vi "Main.vi"() -> ()   [LabVIEW 2013] (continued)
                    n2203 = call "Msgbox - Message Handler.vi"("Short Description (When DB Not Available)"="WPS Details Incomplete" ("string"), "Description (When DB Not Available)"=" must be entered" ("string"), "Pre-Description"=w3600, "<.?....> Message Code"="<E 524>") -> ("MHandler Error"=w3599:errorcluster)  [unwired: 5 in, 2 out]
                    n2204 = local write "MHandler"(w3599) -> ()
                  }
                }
              }
            }
          }
          frame True {
            # "Incomplete Fields In Header"
            n2205 = control-ref of="WPS Details Master Data"() -> (w3634:refnum<vi>)
            n2206 = property class="Clust (strict)"(reference=w3634) -> ("Caption.Text"=w3630:string)  [unwired: 1 in, 2 out]
            n2207 = case shown="\"Master Data Delete\", Default" w3633 {
              tunnel: ["{Delete WPS}" ("string") "{Save WPS}" ("string")] -> _
              frame "Master Data Delete", Default {
                # "No longer available"
              }
              frame "Master Data Save" {
              }
            }
            n2208 = local read "Logon Extra"() -> (w3628:T25)
            n2209 = Unbundle By Name(w3628) -> ("IsUnicode"=w3627:bool)
            n2210 = call "String - Add BOM if IsUnicode.vi"("Input is Unicode (varbinary)?"=w3627, "String IN"=w3630) -> ("BOM Added"=w3629:string)  [unwired: 9 in]
            n2211 = call "Msgbox - Message Handler.vi"("Short Description (When DB Not Available)"=" WPS Details Incomplete", "Description (When DB Not Available)"=" must be entered." ("message"), "Pre-Description"=w3629, "<.?....> Message Code"="<E 524>") -> ("MHandler Error"=w3632:errorcluster)  [unwired: 5 in, 2 out]
            n2212 = local write "MHandler"(w3632) -> ()
          }
        }
      }
      event Mouse Down? {
        # "User Clicks on MasterData\\WPS ComboBox"
        n2213 = event-data() -> ("Time"=→"WPS Details Master Data: Mouse Down":u32, "CtlRef"=w3639:refnum<vi>)  [unwired: 1 in, 6 out]
        n2214 = case shown="True" "DB - Master Data Load" {
          tunnel: w3639 -> [w3642 w3646]
          frame False {
            # "List of wps found"
            # "<wps/ref>_<rev>.wps"
            # "<wps/ref>_<rev>.wps"
            # "Use .wps"
            n2215 = local read "MasterData\\WPS"() -> (w3645:path)
            n2216 = List Folder(path=w3645, pattern="*.wps") -> (filenames=w3641:string[])  [unwired: 2 in, 3 out]
            "Temp Array" <- w3641
            n2217 = call "String - Extract Unique Headers_.vi"("Array In"=w3641) -> ("Array Out"=w3643:string[])  [unwired: 10 in]
            n2218 = property class="CmbBox (strict)"(reference=w3642, "Strings[]"=w3643) -> ()  [unwired: 1 in, 2 out]
          }
          frame True {
            # "Use DB"
            n2219 = call "DB - [MasterData].[Procedure].vi"("DB - Master Data Enum"=DB_-_Master_Data_Procedure_Enum."SELECT [ProcedureNo]", "CmbBox Refnum"=w3646) -> ("SUMMARY"=w3647:errorcluster)  [unwired: 10 in, 3 out]
            n2220 = local write "DB"(w3647) -> ()
          }
        }
        n2221 = event-data() -> ()  [unwired: 2 in, 1 out]
      }
      event Value Change {
        # "<wps/ref>_<rev>.wps"
        n2222 = event-data() -> ("Time"=→"WPS Details Master Data: Value Change":u32, "CtlRef"=w3651:refnum<vi>)  [unwired: 1 in, 4 out]
        n2223 = local read "DB - Master Data Load"() -> (w3653:bool)
        n2224 = property class="CmbBox (strict)"(reference=w3651) -> ("Label.Text"=w3656:string, "Value"=w3654:T5)  [unwired: 1 in, 2 out]
        n2225 = case shown="\"WPS/Ref\", Default" w3656 {
          tunnel: [w3678 w3686 _] -> _
          tunnel: [w3677 w3685 _] -> _
          tunnel: [w3676 w3684 w3697] -> w3655
          tunnel: [w3675 w3683 _] -> _
          tunnel: w3654 -> [w3673 _ w3695]
          tunnel: [w3671 w3682 w3688] -> w3650
          tunnel: [w3670 w3681 w3687] -> w3649
          frame "WPS/Ref", Default {
            w3670 = FALSE  # Include Inactive
            # "Copies Value to Extra WPS\nHighlight Entire Text"
            n2226 = control-ref of="WPS Details Setup"() -> (w3671:refnum<vi>)
            n2227 = control-ref of="WPS/Ref"() -> ()  [unwired: 1 out]
            n2228 = control-ref of="Rev"() -> (w3676:refnum<vi>)
            n2229 = control-ref of="Hold Temperature"() -> (w3677:refnum<vi>)
            n2230 = control-ref of="Hold Time (HH:MM)"() -> (w3675:refnum<vi>)
            n2231 = control-ref of="MCListBox FHS Setup"() -> (w3678:refnum<vi>)
            n2232 = control-ref of="Extra WPS"() -> (w3674:refnum<vi>)
            n2233 = property on="Property Node" class="Str"(reference=w3674, "Value"=w3673) -> (error out=w3672:errorcluster)  [unwired: 1 in, 1 out]
            n2234 = flat-sequence {
              tunnel: w3672 -> [_]
              frame #0 {
                n2235 = property on="Extra WPS" class="Str"("Key Focus"=TRUE, "Text.Selection"=T58 {"Selection Start"=0, "Selection End"=100}) -> ()  [unwired: 2 in, 2 out]
              }
            }
          }
          frame "Master Data WPS/Ref" {
            w3681 = TRUE  # Include Inactive
            n2236 = control-ref of="WPS Details Master Data"() -> (w3682:refnum<vi>)
            n2237 = control-ref of="Master Data WPS/Ref"() -> ()  [unwired: 1 out]
            n2238 = control-ref of="Master Data Rev"() -> (w3684:refnum<vi>)
            n2239 = control-ref of="Master Data Hold Temperature"() -> (w3685:refnum<vi>)
            n2240 = control-ref of="Master Data Hold Time (HH:MM)"() -> (w3683:refnum<vi>)
            n2241 = control-ref of="MCListBox FHS Master Data"() -> (w3686:refnum<vi>)
          }
          frame "Additional WPS/Ref" {
            w3687 = FALSE  # Include Inactive
            w3696 = T13 {"Master Data WPS/Ref"="", "Master Data Rev"="", "Master Data Hold Temperature"="", "Master Data Temperature Units"="", "Master Data Hold Time (HH:MM)"="", "Inactive"=FALSE}  # Cluster
            # "to be implemented"
            n2242 = control-ref of="Additional Rev"() -> (w3697:refnum<vi>)
            n2243 = Bundle(cluster=w3696, "Master Data WPS/Ref"=w3695, "Master Data Rev"=T5 "", "Master Data Hold Temperature"="", "Master Data Temperature Units"="", "Master Data Hold Time (HH:MM)"="", "Inactive"=FALSE) -> (→"WPS Details Buffer (DB)":T13)
            n2244 = control-ref of="WPS Details Buffer (DB)"() -> (w3688:refnum<vi>)
          }
        }
        n2245 = case shown="True" w3653 {
          tunnel: w3655 -> [w3659 w3667]
          tunnel: w3654 -> [w3657 _]
          tunnel: w3650 -> [_ w3664]
          tunnel: w3649 -> [_ w3665]
          frame False {
            # "Show BLANK as Rev and update Details according to BLANK"
            n2246 = local read "Temp Array"() -> (w3661:string[])
            n2247 = call "String - Extract _Body_.vi"("Temp Array"=w3661, "<wps>"=w3657) -> ("<rev>"=w3660:string[])  [unwired: 9 in]
            n2248 = property on="Property Node" class="CmbBox (strict)"(reference=w3659, "Strings[]"=w3660, "Val(Sgnl)"="") -> ()  [unwired: 1 in, 2 out]
          }
          frame True {
            # "This always forces Rev to use \"<Blank>\"\nWhat if Rev  = \"<Blank>\" is Inactive? It will still be loaded.\n\nShould we load the next available one or not load if \"<Blank>\" is inactive"
            # "Destination: WPS Rev ComboBox"
            # "Source: WPS Details Cluster"
            # "Use DB"
            n2249 = call "DB - [MasterData].[Procedure].vi"("DB - Master Data Enum"=DB_-_Master_Data_Procedure_Enum."SELECT [ProcedureRev]", "Include Inactive"=w3665, "Clust Refnum"=w3664, "CmbBox Refnum"=w3667) -> ("Result"=w3662:string[], "SUMMARY"=w3663:errorcluster)  [unwired: 8 in, 2 out]
            n2250 = local write "DB"(w3663) -> ()
            n2251 = disable-structure shown="Disabled" {
              disable-tunnel: w3662 -> [w3669 _]
              frame Disabled {
                # "Rev list"
                n2252 = Index Array(array=w3669) -> ()  [unwired: 1 in, 1 out]
              }
              frame Enabled {
              }
            }
            n2253 = property on="Property Node" class="CmbBox (strict)"(reference=w3667, "Val(Sgnl)"="") -> ()  [unwired: 1 in, 2 out]
          }
        }
      }
      event Value Change {
        # "The [Section] in the .wps file is stored with the Original Ctls Label.Text"
        # "<wps/ref>_<rev>.wps"
        n2254 = event-data() -> ("CtlRef"=w3717:refnum<vi>)  [unwired: 1 in, 5 out]
        n2255 = local read "DB - Master Data Load"() -> (w3705:bool)
        n2256 = property class="CmbBox (strict)"(reference=w3717) -> ("Label.Text"=w3702:string, "Value"=w3708:T5)  [unwired: 1 in, 2 out]
        n2257 = case shown="\"Rev\", Default" w3702 {
          tunnel: [w3744 w3762] -> w3716
          tunnel: [w3752 w3761] -> w3704
          tunnel: [w3751 w3764] -> w3710
          tunnel: [w3750 w3763] -> w3709
          tunnel: [w3749 w3757] -> w3701
          tunnel: [w3748 w3760] -> w3699
          tunnel: w3708 -> [w3745 _]
          tunnel: [w3741 w3759] -> w3707
          tunnel: [w3743 w3758] -> w3706
          tunnel: [w3737 w3756] -> w3698
          frame "Rev", Default {
            w3737 = FALSE  # Include Inactive
            # "Cannot use WPS Details Setup\nbecuase it has extra fields\ncompared to WPS Details Master"
            # "Copies Value to Extra WPS\nHighlight Entire Text"
            n2258 = control-ref of="WPS Details Temperature Units"() -> (w3748:refnum<vi>)
            n2259 = local read "Setup Edit"() -> (w3740:bool)
            n2260 = control-ref of="WPS Details Setup"() -> (w3749:refnum<vi>)
            n2261 = control-ref of="WPS/Ref"() -> (w3744:refnum<vi>)
            n2262 = control-ref of="Rev"() -> ()  [unwired: 1 out]
            n2263 = control-ref of="Hold Temperature"() -> (w3751:refnum<vi>)
            n2264 = control-ref of="Hold Time (HH:MM)"() -> (w3750:refnum<vi>)
            n2265 = control-ref of="MCListBox FHS Setup"() -> (w3752:refnum<vi>)
            n2266 = local read "CellBG Unused Cells"() -> (w3741:u32)
            n2267 = local read "Edit WPS in Setup"() -> (w3739:bool)
            n2268 = control-ref of="Extra Rev"() -> (w3746:refnum<vi>)
            n2269 = property on="Property Node" class="Str"(reference=w3746, "Value"=w3745) -> (error out=w3747:errorcluster)  [unwired: 1 in, 1 out]
            n2270 = And(x=w3740, y=w3739) -> (x .and. y?=w3738:bool)
            n2271 = local read "CellBG New Cells"() -> (w3742:u32)
            n2272 = disable-structure shown="Disabled" {
              disable-tunnel: w3747 -> [w3753 _]
              frame Disabled {
                n2273 = flat-sequence {
                  tunnel: w3753 -> [_]
                  frame #0 {
                    n2274 = property on="Extra Rev" class="Str"("Key Focus"=TRUE, "Text.Selection"=T58 {"Selection Start"=0, "Selection End"=100}) -> ()  [unwired: 2 in, 2 out]
                  }
                }
              }
              frame Enabled {
              }
            }
            n2275 = Select(t=w3742, s=w3738, f=w3741) -> (s? t:f=w3743:u32)
          }
          frame "Master Data Rev" {
            w3756 = TRUE  # Include Inactive
            n2276 = control-ref of="Master Data Temperature Units"() -> (w3760:refnum<vi>)
            n2277 = control-ref of="WPS Details Master Data"() -> (w3757:refnum<vi>)
            n2278 = control-ref of="Master Data WPS/Ref"() -> (w3762:refnum<vi>)
            n2279 = control-ref of="Master Data Rev"() -> ()  [unwired: 1 out]
            n2280 = control-ref of="Master Data Hold Temperature"() -> (w3764:refnum<vi>)
            n2281 = control-ref of="Master Data Hold Time (HH:MM)"() -> (w3763:refnum<vi>)
            n2282 = control-ref of="MCListBox FHS Master Data"() -> (w3761:refnum<vi>)
            n2283 = local read "CellBG Unused Cells"() -> (w3759:u32)
            n2284 = local read "CellBG New Cells"() -> (w3758:u32)
          }
        }
        n2285 = property on="Property Node" class="CmbBox (strict)"(reference=w3716) -> ("Value"=w3713:T5)  [unwired: 1 in, 2 out]
        n2286 = case shown="True" w3705 {
          tunnel: w3713 -> [w3725 _]
          tunnel: [w3721 _] -> w3712
          tunnel: [w3720 w3733] -> w3711
          tunnel: w3708 -> [w3719 _]
          tunnel: w3701 -> [_ w3730]
          tunnel: w3704 -> [_ w3731]
          tunnel: [_ w3732] -> w3703
          tunnel: [w3718 w3729] -> w3700
          tunnel: w3698 -> [_ w3728]
          frame False {
            n2287 = Concatenate Strings(w3725, "_" ("string"), w3719, ".wps" ("string")) -> (w3723:string)
            n2288 = local read "MasterData\\WPS"() -> (w3722:path)
            n2289 = Build Path(base path=w3722, name or relative path=w3723) -> (appended path=w3726:path)
            n2290 = call <vilib>:"Check if File or Folder Exists.vi"("path"=w3726) -> ("error out"=w3718:errorcluster, "file or folder exists?"=w3720:bool, "dup path"=w3721:path)  [unwired: 8 in]
          }
          frame True {
            # "At least 1 Record"
            # "Use DB"
            n2291 = call "DB - [MasterData].[Procedure].vi"("DB - Master Data Enum"=DB_-_Master_Data_Procedure_Enum."SELECT [MasterData].[ProcedureItem]", "Include Inactive"=w3728, "MCListbox Refnum"=w3731, "Clust Refnum"=w3730) -> ("ItemNames"=w3735:string[][], "SUMMARY"=w3729:errorcluster)  [unwired: 8 in, 2 out]
            n2292 = Array Size(array=w3735) -> (size(s)=w3732:i32[])
            n2293 = Index Array(array=w3732) -> (element=w3734:i32)  [unwired: 1 in]
            n2294 = local write "DB"(w3729) -> ()
            n2295 = Greater Than 0?(x=w3734) -> (x > 0?=w3733:bool)
          }
        }
        n2296 = control-ref of="MCListBox FHS Master Data"() -> (w3715:refnum<vi>)
        n2297 = control-ref of="WPS Details Master Data"() -> (w3714:refnum<vi>)
        n2298 = case shown="True" w3711 {
          tunnel: w3712 -> [_ w3796]
          tunnel: w3701 -> [_ w3789]
          tunnel: w3704 -> [w3774 w3786]
          tunnel: w3714 -> [_ w3788]
          tunnel: w3715 -> [_ w3787]
          tunnel: w3710 -> [w3773 _]
          tunnel: w3709 -> [w3772 _]
          tunnel: w3707 -> [w3770 w3785]
          tunnel: w3706 -> [w3769 w3784]
          tunnel: w3705 -> [_ w3783]
          tunnel: w3703 -> [_ w3782]
          tunnel: w3700 -> [_ _]
          tunnel: w3699 -> [w3767 _]
          frame False {
            w3771 = "" ("Value")
            w3776 = 4 ("dimension size")
            # "<wps/ref>_.wps does not exisit"
            # "DB/File no record"
            n2299 = property on="Master Data Temperature Units / WPS Details Temperature Units" class="Str"(reference=w3767) -> (reference out=w3765:refnum<vi>, "Label.Text"=w3766:string)  [unwired: 1 in, 1 out]
            n2300 = Initialize Array("", w3776) -> (w3779:string[])
            n2301 = Build Array(w3779) -> (w3778:string[][])
            n2302 = case shown="\"Master Data Temperature Units\"" w3766 {
              tunnel: w3765 -> [_ w3781]
              frame "False", Default {
              }
              frame "Master Data Temperature Units" {
                # "New Master Data, we default to Global Temperature Units,\notherwise it will be blank if user Enters a new MasterData Ref or Rev"
                n2303 = global read "Global SRTRS.vi" "Temperature Units"() -> (w3780:string)
                n2304 = property on="Master Data Temperature Units" class="Str"(reference=w3781, "Text.Text"=w3780) -> ()  [unwired: 1 in, 2 out]
              }
            }
            n2305 = property on="Property Node" class="MCListbox (strict)"(reference=w3774, "ItemNames"=w3778, "NumCols"=w3776) -> (reference out=w3775:refnum<vi>)  [unwired: 1 in, 1 out]
            n2306 = property on="Master Data Hold Temperature / Hold Temperature" class="Str"(reference=w3773, "Value"=w3771) -> ()  [unwired: 1 in, 2 out]
            n2307 = property on="Master Data Hold Time / Hold Time" class="Str"(reference=w3772, "Value"=w3771) -> ()  [unwired: 1 in, 2 out]
            n2308 = call "MCListbox Refresh.vi"("Which Cells"=T46."Exisiting and Blank Cells", "color of New Cells"=w3769, "color of Blank cells"=w3770, "MulticolumnListbox in"=w3775) -> ()  [unwired: 6 in, 2 out]
          }
          frame True {
            # "DB/File Exisits"
            n2309 = case shown="True" w3783 {
              tunnel: w3796 -> [w3804 _]
              tunnel: [w3803 w3811] -> w3794
              tunnel: [w3802 _] -> w3791
              tunnel: w3789 -> [w3801 _]
              tunnel: w3788 -> [w3800 _]
              tunnel: w3787 -> [w3799 _]
              tunnel: w3786 -> [w3798 _]
              tunnel: w3782 -> [_ w3811]
              frame False {
                n2310 = call <vilib>:"Open Config Data.vi"("create file if necessary (T)"=FALSE, "configuration file path"=w3804) -> ("error out"=w3809:errorcluster, "refnum"=w3810:T59)  [unwired: 7 in, 1 out]
                n2311 = call "Key - Cluster Read.vi"("error in (no error)"=w3809, "New Ctl Ref"=w3801, "Original Ctl Ref"=w3800, "Refnum in"=w3810) -> ("error out"=w3808:errorcluster, "Refnum out"=w3807:T59)  [unwired: 5 in, 1 out]
                n2312 = call "Key - MCListbox Read.vi"("error in (no error)"=w3808, "New MulticolumnListbox Ref"=w3798, "Original MulticolumnListbox Ref"=w3799, "refnum"=w3807) -> ("error out"=w3806:errorcluster, "size(s)"=w3803:i32[], "Refnum out"=w3805:T59)  [unwired: 4 in, 1 out]
                n2313 = call <vilib>:"Close Config Data.vi"("error in (no error)"=w3806, "refnum"=w3805) -> ("error out"=w3802:errorcluster)  [unwired: 8 in, 1 out]
              }
              frame True {
                # "Use DB"
              }
            }
            n2314 = Add Array Elements(numeric array=w3794) -> (sum=w3793:i32)
            n2315 = case shown="0" w3793 {
              tunnel: w3786 -> [w3813 w3817]
              tunnel: [w3813 w3816] -> w3792
              tunnel: w3791 -> [w3812 w3815]
              tunnel: [w3812 w3814] -> w3790
              frame 1, Default {
              }
              frame 0 {
                w3821 = 4 ("dimension size")
                # "Minimum 1 row"
                n2316 = Initialize Array("", w3821) -> (w3819:string[])
                n2317 = Build Array(w3819) -> (w3818:string[][])
                n2318 = property on="Property Node" class="MCListbox (strict)"(reference=w3817, error in=w3815, "ItemNames"=w3818, "NumCols"=w3821) -> (reference out=w3816:refnum<vi>, error out=w3814:errorcluster)
              }
            }
            n2319 = call "MCListbox Refresh.vi"("Which Cells"=T46."Exisiting and Blank Cells", "Error In"=w3790, "color of New Cells"=w3784, "color of Blank cells"=w3785, "MulticolumnListbox in"=w3792) -> ()  [unwired: 5 in, 2 out]
          }
        }
      }
      event "WPS Details Master Data.Master Data Hold Temperature", "WPS Details Master Data.Master Data Hold Time (HH:MM)", "WPS Details Setup.Hold Temperature", "WPS Details Setup.Hold Time (HH:MM)": Value Change {
        n2320 = event-data() -> ("CtlRef"=w3826:refnum<vi>, "NewVal"=w3824:string)  [unwired: 1 in, 4 out]
        n2321 = property class="Str"(reference=w3826) -> (reference out=w3823:refnum<vi>, "Label.Text"=w3825:string)  [unwired: 1 in, 1 out]
        n2322 = case shown="\"Hold Temperature\", \"Master Data Hold Temperature\"" w3825 {
          tunnel: w3824 -> [w3827 w3834]
          tunnel: [w3828 w3833] -> w3822
          frame "False", Default {
            # "Formats String to (HH:SS)"
            n2323 = call "String - Format to (HH_colon_MM).vi"("xx:xx"=w3827) -> ("(HH:mm)"=w3828:string)  [unwired: 9 in, 1 out]
          }
          frame "Hold Temperature", "Master Data Hold Temperature" {
            n2324 = Decimal String To Number(string=w3834) -> (number=w3832:i32)  [unwired: 2 in, 1 out]
            n2325 = In Range and Coerce(upper limit=1000 ("y"), x=w3832, lower limit=23 ("x")) -> (coerced(x)=w3829:i32)  [unwired: 1 out]
            n2326 = Number To Decimal String(number=w3829) -> (decimal integer string=w3833:string)  [unwired: 1 in]
          }
        }
        n2327 = property class="Str"(reference=w3823, "Value"=w3822) -> ()  [unwired: 1 in, 2 out]
      }
      event "WPS Details Setup.Hold Temperature", "WPS Details Setup.Hold Time (HH:MM)", "WPS Details Master Data.Master Data Hold Temperature", "WPS Details Master Data.Master Data Hold Time (HH:MM)": Key Down? {
        n2328 = event-data() -> ("Char"=w3836:i16, "VKey"=w3835:T55)  [unwired: 1 in, 8 out]
        n2329 = case "Only NUMBERS, colon, BackSpace, TAB, (Enter, Return, Up, Down, Right, Left, Delete)" shown="8, 9, 48..58" w3836 {
          tunnel: [w3839 w3842] -> w3837
          tunnel: w3835 -> [w3838 _]
          frame 0, Default {
            # "Exception"
            n2330 = case shown="Default" w3838 {
              tunnel: [w3840 w3841] -> w3839
              frame Default {
                w3840 = TRUE  # Discard
              }
              frame "Enter", "Return", "Up".."Right", "Delete" {
                w3841 = FALSE  # Do Not Discard
                # "Up, Down, Left, Right, Delete"
              }
            }
          }
          frame 8, 9, 48..58 {
            w3842 = FALSE  # Do not discard
            # "Char\n46        .     (decimal Point)\n48-57  0-9 (Numbers)\n58        :      (colon)\n8          Backspace\n9          TAB"
            # "Backspace, TAB, Numbers, colon"
          }
        }
        n2331 = event-data("Discard?"=w3837) -> ()  [unwired: 1 in, 1 out]
      }
      event "WPS Details Setup.Hold Temperature", "WPS Details Setup.Hold Time (HH:MM)", "WPS Details Master Data.Master Data Hold Temperature", "WPS Details Master Data.Master Data Hold Time (HH:MM)": Key Down {
        # "All controls in the same cluster has same OwningPane"
        n2332 = event-data() -> ("CtlRef"=w3847:refnum<vi>, "Char"=w3849:i16, "VKey"=w3848:T55)  [unwired: 1 in, 7 out]
        n2333 = property on="Hold Temperature" class="Str"() -> ("OwningPane"=w3843:refnum<vi>)  [unwired: 2 in, 2 out]
        n2334 = property class="Str"(reference=w3847) -> ("OwningPane"=w3846:refnum<vi>)  [unwired: 1 in, 2 out]
        n2335 = case shown="\"ASCII\", Default" w3848 {
          tunnel: w3849 -> [w3886 _]
          tunnel: [w3885 TRUE] -> w3850
          frame "ASCII", Default {
            n2336 = Equal?(x=w3886, y=i16 9) -> (x = y?=w3885:bool)
          }
          frame "Enter", "Return" {
          }
        }
        n2337 = Equal?(x=w3843, y=w3846) -> (x = y?=w3845:bool)
        n2338 = case shown="True" w3845 {
          tunnel: [w3883 w3884] -> w3844
          frame False {
            n2339 = control-ref of="WPS Details Master Data"() -> (w3883:refnum<vi>)
          }
          frame True {
            n2340 = control-ref of="WPS Details Setup"() -> (w3884:refnum<vi>)
          }
        }
        n2341 = case shown="True" w3850 {
          tunnel: w3847 -> [_ w3857]
          tunnel: w3844 -> [_ w3853]
          frame False {
          }
          frame True {
            n2342 = property class="Clust (strict)"(reference=w3853) -> ("Controls[]"=w3855:refnum<vi>[])  [unwired: 1 in, 2 out]
            n2343 = Search 1D Array(1D array=w3855, element=w3857) -> (index of element=w3860:i32)  [unwired: 1 in]
            n2344 = property class="Str"(reference=w3857) -> (reference out=w3859:refnum<vi>, "Label.Text"=w3858:string, "Value"=w3851:string)  [unwired: 1 in, 1 out]
            n2345 = Increment(x=w3860) -> (x+1=w3854:i32)
            n2346 = case shown="\"Rev\"" w3858 {
              tunnel: w3859 -> [w3862 _ _ _]
              tunnel: [w3869 w3873 w3877 w3880] -> w3856
              tunnel: w3855 -> [w3871 w3875 w3879 w3882]
              tunnel: w3854 -> [w3870 _ w3878 _]
              tunnel: [TRUE ("Key Focus") TRUE ("Key Focus") TRUE ("Key Focus") _] -> w3852
              tunnel: w3851 -> [w3863 _ _ _]
              frame "Hold Temperature", "Master Data Hold Temperature" {
                # "Min 25 degC, SKIP Temperature Units"
                n2347 = Decimal String To Number(string=w3863) -> (number=w3866:i32)  [unwired: 2 in, 1 out]
                n2348 = Max & Min(x=23, y=w3866) -> (max(x,y)=w3864:i32)  [unwired: 1 out]
                n2349 = Number To Decimal String(number=w3864) -> (decimal integer string=w3861:string)  [unwired: 1 in]
                n2350 = property class="Str"(reference=w3862, "Value"=w3861) -> ()  [unwired: 1 in, 2 out]
                n2351 = Increment(x=w3870) -> (x+1=w3867:i32)
                n2352 = Index Array(array=w3871, index=w3867) -> (element=w3869:refnum<vi>)
              }
              frame "Rev" {
                # "Because of extra 2 fields in WPS cluster of SETUP. We cannot \nreorder or it will affect the Key- Cluster Write"
                # "Goto WPS"
                n2353 = Index Array(array=w3875, index=5) -> (element=w3873:refnum<vi>)
              }
              frame Default {
                # "TAB to next"
                n2354 = Index Array(array=w3879, index=w3878) -> (element=w3877:refnum<vi>)
              }
              frame "Hold Time (HH:MM)", "Master Data Hold Time (HH:MM)" {
                # "Last"
                n2355 = Index Array(array=w3882, index=0) -> (element=w3880:refnum<vi>)
              }
            }
            n2356 = property class="Ctl"(reference=w3856, "Key Focus"=w3852) -> ()  [unwired: 1 in, 2 out]
          }
        }
      }
      event "Extra WPS", "Extra Rev": Key Down {
        # "All controls in the same cluster has same OwningPane"
        n2357 = event-data() -> ("CtlRef"=w3889:refnum<vi>, "Char"=w3891:i16, "VKey"=w3890:T55)  [unwired: 1 in, 7 out]
        n2358 = case shown="\"ASCII\", Default" w3890 {
          tunnel: w3891 -> [w3904 _]
          tunnel: [w3903 TRUE] -> w3892
          frame "ASCII", Default {
            n2359 = Equal?(x=w3904, y=i16 9) -> (x = y?=w3903:bool)
          }
          frame "Enter", "Return" {
          }
        }
        n2360 = case shown="True" w3892 {
          tunnel: w3889 -> [_ w3896]
          frame False {
          }
          frame True {
            n2361 = property class="Str"(reference=w3896) -> (reference out=w3898:refnum<vi>, "Label.Text"=w3897:string, "Value"=w3893:string)  [unwired: 1 in, 1 out]
            n2362 = case shown="\"Extra WPS\", Default" w3897 {
              tunnel: w3898 -> [_ _]
              tunnel: [w3899 w3902] -> w3895
              tunnel: [TRUE ("Key Focus") TRUE ("Key Focus")] -> w3894
              tunnel: w3893 -> [_ _]
              frame "Extra WPS", Default {
                # "Because of extra 2 fields in cluster. We cannot \nreorder or it will affect the Key- Cluster Write"
                # "Goto Hold Tempeterature"
                n2363 = control-ref of="Extra Rev"() -> (w3899:refnum<vi>)
              }
              frame "Extra Rev" {
                n2364 = control-ref of="Hold Temperature"() -> (w3902:refnum<vi>)
              }
            }
            n2365 = property class="Str"(reference=w3895, "Key Focus"=w3894) -> ()  [unwired: 1 in, 2 out]
          }
        }
      }
      event "WPS Details Master Data.Inactive": Value Change {
        n2366 = event-data() -> ("NewVal"=w3907:bool)  [unwired: 1 in, 5 out]
        n2367 = case shown="True" w3907 {
          frame False {
          }
          frame True {
            n2368 = property on="Master Data Rev" class="CmbBox (strict)"() -> ("Value"=w3911:T5)  [unwired: 2 in, 2 out]
            n2369 = property on="Master Data WPS/Ref" class="CmbBox (strict)"() -> ("Value"=w3912:T5)  [unwired: 2 in, 2 out]
            n2370 = call "String - Create comma seperated String.vi"("B"=w3911, "A"=w3912) -> ("A, B , C (auto comma)"=w3910:string)  [unwired: 9 in]
            n2371 = call "Msgbox - Message Handler.vi"("Short Description (When DB Not Available)"="Inactive WPS", "Description (When DB Not Available)"=" cannot be used after inactive. Do you wish to proceed?", "Pre-Description"=w3910, "<.?....> Message Code"="<W 523>") -> ("MHandler Error"=w3908:errorcluster, "OK Out"=w3909:bool)  [unwired: 5 in, 1 out]
            n2372 = local write "MHandler"(w3908) -> ()
            n2373 = property on="Inactive" class="Bool (strict)"("Value"=w3909) -> ()  [unwired: 2 in, 2 out]
          }
        }
      }
      event "---------------------------------       Master Data (Material)      -----------------------------": Value Change {
        n2374 = event-data() -> ()  [unwired: 1 in, 6 out]
      }
      event "Material New": Value Change {
        # "MasterData Material"
        n2375 = event-data() -> ()  [unwired: 1 in, 6 out]
        n2376 = call "Msgbox - Message Handler.vi"("Short Description (When DB Not Available)"="Create New Material", "Description (When DB Not Available)"="All unsaved data will be lost. Do you want to proceed?", "<.?....> Message Code"="<W 501>") -> ("MHandler Error"=w3920:errorcluster, "OK Out"=w3919:bool)  [unwired: 6 in, 1 out]
        n2377 = local write "MHandler"(w3920) -> ()
        n2378 = case shown="True" w3919 {
          frame False {
          }
          frame True {
            w3921 = T30."Disabled and Grayed Out" ("Disabled")
            w3924 = ""
            n2379 = control-ref of="Master Data Thermocouple Location"() -> (w3922:refnum<vi>)
            n2380 = control-ref of="Master Data Material Description"() -> (w3925:refnum<vi>)
            n2381 = invoke class="Pict" method="Reinit To Default"(reference=w3922) -> ()  [unwired: 2 in, 3 out]
            n2382 = invoke class="Str" method="Reinit To Default"(reference=w3925) -> ()  [unwired: 2 in, 3 out]
            n2383 = property on="Material Copy" class="Bool"("DisabledEnum"=w3921) -> ()  [unwired: 2 in, 2 out]
            n2384 = property on="SAPMaterial Description (Long) Master Data Tab" class="Bool"("DisabledEnum"=w3921) -> ()  [unwired: 2 in, 2 out]
            n2385 = property on="Material Save" class="Bool"("DisabledEnum"=w3921) -> ()  [unwired: 2 in, 2 out]
            n2386 = property on="Master Data Material" class="CmbBox"("Value"=w3924) -> ()  [unwired: 2 in, 2 out]
            n2387 = property on="Master Data Rev" class="CmbBox"("Value"=w3924, "Strings[]"=string[] [] ("Strings []")) -> ()  [unwired: 2 in, 2 out]
          }
        }
      }
      event "Material Save", "Material Delete": Value Change {
        # "<material>_<rev>_<description>.jpg"
        # "{Save Material}/{Delete Material}"
        n2388 = event-data() -> ("CtlRef"=w3932:refnum<vi>)  [unwired: 1 in, 5 out]
        n2389 = Unbundle By Name("Material") -> ("Master Data Material"=w3928:string, "Master Data Rev"=w3927:string, "Master Data Material Description"=w3929:string)
        n2390 = property class="Bool"(reference=w3932) -> ("Label.Text"=w3931:string)  [unwired: 1 in, 2 out]
        n2391 = Empty String/Path?(string/path=w3928) -> (empty?=w3926:bool)
        n2392 = case shown="False" w3926 {
          tunnel: w3931 -> [w3944 _]
          tunnel: [w3940 _] -> _
          tunnel: w3929 -> [w3939 _]
          tunnel: w3928 -> [w3935 w4096]
          tunnel: w3927 -> [w3934 w4095]
          frame False {
            w3943 = "_"
            # "Valid Fields"
            n2393 = local read "MasterData Image File Path"() -> (w3942:path)
            n2394 = Concatenate Strings(w3935, w3943, w3934, w3943) -> (w3936:string)
            n2395 = local read "MasterData\\JPG"() -> (w3937:path)
            n2396 = Concatenate Strings(w3936, w3939, ".jpg" ("string")) -> (w3933:string)
            n2397 = Build Path(base path=w3937, name or relative path=w3933) -> (appended path=w3941:path)
            n2398 = case shown="\"Material Save\"" w3944 {
              tunnel: w3942 -> [_ w3997]
              tunnel: w3941 -> [w3949 w3994]
              tunnel: [w3945 w3992] -> w3940
              tunnel: w3937 -> [_ w3995]
              tunnel: w3936 -> [_ w3996]
              tunnel: w3933 -> [_ _]
              frame "Material Delete", Default {
                n2399 = Delete(path (use dialog)=w3949, confirm (F)=TRUE) -> (cancelled=w3950:bool, error out=w3948:errorcluster)  [unwired: 3 in, 1 out]
                n2400 = case shown="False" w3950 {
                  tunnel: w3949 -> [w3957 _]
                  tunnel: [w3954 _] -> w3945
                  tunnel: [w3956 "{Delete Material} Cancelled By User." ("string")] -> w3946
                  tunnel: [TRUE FALSE] -> w3947
                  tunnel: w3948 -> [w3954 _]
                  frame False {
                    n2401 = control-ref of="Master Data Material Description"() -> (w3959:refnum<vi>)
                    n2402 = control-ref of="Master Data Thermocouple Location"() -> (w3960:refnum<vi>)
                    n2403 = invoke class="Pict" method="Reinit To Default"(reference=w3960) -> ()  [unwired: 2 in, 3 out]
                    n2404 = invoke class="Str" method="Reinit To Default"(reference=w3959) -> ()  [unwired: 2 in, 3 out]
                    n2405 = case shown="No Error" w3954 {
                      tunnel: w3957 -> [w3969 _]
                      tunnel: [w3965 w3972] -> w3956
                      tunnel: "{Delete Material}" ("string") -> [w3963 w3971]
                      frame No Error {
                        w3967 = "\"" ("string")
                        # "File Delete OK"
                        n2406 = Path To String(path=w3969) -> (string=w3968:string)
                        n2407 = Concatenate Strings(w3963, " OK." ("string"), "\n") -> (w3962:string)
                        n2408 = Concatenate Strings(w3962, w3967, w3968, w3967, " deleted. " ("string")) -> (w3965:string)
                      }
                      frame Error {
                        # "File Delete Failed"
                        n2409 = Concatenate Strings(w3971, " Not OK.", "\n") -> (w3972:string)
                      }
                    }
                  }
                  frame True {
                  }
                }
                n2410 = case shown="True" w3947 {
                  tunnel: w3946 -> [_ w3953]
                  tunnel: w3945 -> [_ _]
                  frame False {
                    # "Delete Cancelled"
                  }
                  frame True {
                    # "Delete OK/Fail"
                    n2411 = call "Queue - EnQueue to MessageQ.vi"("<NoD> Don't Display to UI"=TRUE, "Message"=w3953) -> ()  [unwired: 9 in, 1 out]
                  }
                }
              }
              frame "Material Save" {
                n2412 = local read "DB - Master Data Save"() -> (w3993:bool)
                n2413 = control-ref of="Material"() -> (w3978:refnum<vi>)
                n2414 = property class="Clust (strict)"(reference=w3978) -> ("Value"=w3979:T12)  [unwired: 1 in, 2 out]
                n2415 = Unbundle By Name(w3979) -> ("Master Data Material"=w3984:string, "Master Data Rev"=w3985:string)
                n2416 = Empty String/Path?(string/path=w3985) -> (empty?=w3983:bool)
                n2417 = Select(t="", s=w3983, f=", " ("string")) -> (s? t:f=w3980:string)
                n2418 = Concatenate Strings(w3984, w3980, w3985) -> (w3976:string)
                n2419 = case shown="True" w3993 {
                  tunnel: w3997 -> [w4019 w4043]
                  tunnel: w3996 -> [w4018 _]
                  tunnel: w3995 -> [w4017 _]
                  tunnel: [w4009 w4039] -> w3992
                  tunnel: w3994 -> [w4003 _]
                  tunnel: [w4008 w4055] -> w3991
                  tunnel: [w4007 w4054] -> w3990
                  tunnel: [w3998 w4053] -> w3989
                  tunnel: [w4006 w4052] -> w3988
                  tunnel: [w4000 w4046] -> w3986
                  tunnel: w3976 -> [w3999 w4044]
                  tunnel: w3978 -> [_ w4042]
                  frame False {
                    w4005 = "\"" ("string")
                    # "Use File IO"
                    n2420 = Concatenate Strings(w4018, "*.*" ("string")) -> (w4011:string)
                    n2421 = List Folder(path=w4017, pattern=w4011) -> (path out=w4013:path, filenames=w4012:string[])  [unwired: 2 in, 2 out]
                    n2422 = for {
                      tunnel: w4013 -> [w4035]
                      tunnel: w4012 -> [w4034] mode=indexing
                      tunnel: [w4033] -> w4015 mode=indexing
                      tunnel: w4003 -> [w4032]
                      # "Delete all other <material>_<rev>_*.*"
                      n2423 = Build Path(base path=w4035, name or relative path=w4034) -> (appended path=w4031:path)
                      n2424 = Not Equal?(x=w4031, y=w4032) -> (x != y?=w4030:bool)
                      n2425 = case shown="True" w4030 {
                        tunnel: [_ w4037] -> w4033
                        tunnel: w4031 -> [_ w4036]
                        frame False {
                        }
                        frame True {
                          n2426 = Delete(path (use dialog)=w4036) -> (error out=w4037:errorcluster)  [unwired: 4 in, 2 out]
                        }
                      }
                    }
                    n2427 = Copy(9:TRUE ("overwrite (F)"), 10:w4003, 11:w4019) -> (0:w4016:errorcluster)  [unwired: 2 in, 2 out]
                    n2428 = Merge Errors(w4016, w4015) -> (w4009:errorcluster)
                    n2429 = case shown="Error" w4009 {
                      tunnel: ["Material Saved" ("string") "Material Save Failed" ("string")] -> w4008
                      tunnel: [" material details saved." ("string") " material details cannot be saved." ("string")] -> w4007
                      tunnel: ["<I 502>" ("string") "<E 505>" ("string")] -> w4006
                      tunnel: ["{Material Save} OK. " ("string") "{Material Save} Failed. " ("string")] -> w4002
                      tunnel: w3999 -> [w4020 w4026]
                      tunnel: [w4020 w4026] -> w3998
                      frame No Error {
                        # "File Save OK"
                      }
                      frame Error {
                        # "File Save Not OK"
                      }
                    }
                    n2430 = Path To String(path=w4003) -> (string=w4004:string)
                    n2431 = Concatenate Strings(w4005, w4004, w4005) -> (w4001:string)
                    n2432 = Concatenate Strings(w4002, w4001) -> (w4000:string)
                  }
                  frame True {
                    w4050 = "\"" ("string")
                    # "Use DB"
                    n2433 = local read "Logon"() -> (w4056:T21)
                    n2434 = Unbundle By Name(w4056) -> ("LanguageID"=w4041:string)
                    n2435 = call "DB - [MasterData].[Material].vi"("DB - Master Data Material Enum"=DB_-_Master_Data_Material_Enum."INSERT [MasterData].[Material]", "[LanguageId]"=w4041, "Clust Refnum"=w4042, "Material File"=w4043) -> ("SUMMARY"=w4040:errorcluster)  [unwired: 7 in, 4 out]
                    n2436 = Unbundle By Name(w4040) -> ("code"=w4045:i32)
                    n2437 = local write "DB"(w4040) -> ()
                    n2438 = case shown="9724" w4045 {
                      tunnel: w4044 -> [_ w4066]
                      tunnel: w4043 -> [_ w4065]
                      tunnel: w4042 -> [_ w4064]
                      tunnel: w4041 -> [_ w4063]
                      tunnel: w4040 -> [w4059 _]
                      tunnel: [w4059 w4061] -> w4039
                      tunnel: [w4058 w4060] -> w4038
                      frame 0, Default {
                        w4058 = TRUE  # INSERT OK
                      }
                      frame 9724 {
                        n2439 = call "Msgbox - Message Handler.vi"("Short Description (When DB Not Available)"="Material Exists", "Description (When DB Not Available)"=" material exists. Do you want to overwrite?" ("Short Description (When DB Not Available)"), "Pre-Description"=w4066, "<.?....> Message Code"="<W 506>" ("string")) -> ("MHandler Error"=w4062:errorcluster, "OK Out"=w4060:bool)  [unwired: 5 in, 1 out]
                        n2440 = local write "MHandler"(w4062) -> ()
                        n2441 = case shown="True" w4060 {
                          tunnel: w4065 -> [_ w4075]
                          tunnel: w4064 -> [_ w4074]
                          tunnel: w4063 -> [_ w4073]
                          tunnel: w4062 -> [w4070 w4072]
                          tunnel: [w4070 w4071] -> w4061
                          frame False {
                          }
                          frame True {
                            n2442 = call "DB - [MasterData].[Material].vi"("DB - Master Data Material Enum"=DB_-_Master_Data_Material_Enum."UPDATE [MasterData].[Material]", "[LanguageId]"=w4073, "error in (no error)"=w4072, "Clust Refnum"=w4074, "Material File"=w4075) -> ("SUMMARY"=w4071:errorcluster)  [unwired: 6 in, 4 out]
                          }
                        }
                      }
                    }
                    n2443 = local write "DB"(w4039) -> ()
                    n2444 = case shown="Error" w4039 {
                      tunnel: [w4082 "Material Save Failed" ("string")] -> w4055
                      tunnel: [w4081 " material details cannot be saved." ("string")] -> w4054
                      tunnel: [w4079 w4091] -> w4053
                      tunnel: [w4080 "<E 505>" ("string")] -> w4052
                      tunnel: w4044 -> [w4079 w4091]
                      tunnel: ["{Material Save} OK. " ("string") "{Material Save} Failed. " ("string")] -> w4047
                      tunnel: w4038 -> [w4077 _]
                      frame No Error {
                        # "DB Update OK"
                        n2445 = case shown="False" w4077 {
                          tunnel: ["Material Saved" ("string") "Material Save Cancelled" ("string")] -> w4082
                          tunnel: [" material details saved." ("string") " material save is cancelled." ("string")] -> w4081
                          tunnel: ["<I 502>" ("string") "<I 507>" ("string")] -> w4080
                          frame True {
                          }
                          frame False {
                            # "Save Cancelled"
                          }
                        }
                      }
                      frame Error {
                        # "DB Update Failed"
                      }
                    }
                    n2446 = Path To String(path=w4043) -> (string=w4051:string)
                    n2447 = Path To String(path=w4043) -> (string=w4048:string)
                    n2448 = Concatenate Strings(w4047, w4050, w4048, w4050, " \nsaved to \n" ("string"), w4050, w4051, w4050) -> (w4046:string)
                  }
                }
                n2449 = call "Queue - EnQueue to MessageQ.vi"("<NoD> Don't Display to UI"=TRUE, "Message"=w3986) -> ()  [unwired: 9 in, 1 out]
                n2450 = call "Msgbox - Message Handler.vi"("Short Description (When DB Not Available)"=w3991, "Description (When DB Not Available)"=w3990, "Pre-Description"=w3989, "<.?....> Message Code"=w3988) -> ("MHandler Error"=w3977:errorcluster)  [unwired: 5 in, 2 out]
                n2451 = local write "MHandler"(w3977) -> ()
              }
            }
          }
          frame True {
            (unwired) "[Save/Delete Material] Some Fields Are Invalid." ("string")
            (unwired) FALSE
            # "Some Fields are empty"
            n2452 = Empty String/Path?(string/path=w4095) -> (empty?=w4100:bool)
            n2453 = Select(t="", s=w4100, f=", " ("string")) -> (s? t:f=w4097:string)
            n2454 = Concatenate Strings(w4096, w4097, w4095) -> (w4094:string)
            n2455 = call "Msgbox - Message Handler.vi"("Short Description (When DB Not Available)"="Material Save Failed" ("string"), "Description (When DB Not Available)"=" material details cannot be saved." ("string"), "Pre-Description"=w4094, "<.?....> Message Code"="<E 505>" ("string")) -> ("MHandler Error"=w4104:errorcluster)  [unwired: 5 in, 2 out]
            n2456 = local write "MHandler"(w4104) -> ()
          }
        }
      }
      event "Material Browse": Value Change {
        n2457 = event-data() -> ()  [unwired: 1 in, 6 out]
        n2458 = local read "MasterData\\JPG"() -> (w4109:path)
        n2459 = call "File Dialog2"("start path"=w4109, "prompt"="Select Material image", "pattern (all files)"="*.jpg;*.jpeg") -> ("selected path"=w4108:path, "exists"=w4107:bool, "error out"=w4106:errorcluster)  [unwired: 9 in, 1 out]
        n2460 = case shown="True" w4107 {
          tunnel: w4108 -> [_ w4113]
          tunnel: w4106 -> [_ _]
          frame False {
          }
          frame True {
            n2461 = call <vilib>:"Read JPEG File.vi"("path to JPEG file"=w4113) -> ("image data"=w4112:T40)  [unwired: 8 in, 2 out]
            n2462 = call <vilib>:"Draw Flattened Pixmap.vi"("image data"=w4112, "picture"=picture data[5B]) -> ("new picture"=→"Master Data Thermocouple Location":picture)  [unwired: 7 in]
            n2463 = disable-structure shown="Disabled" {
              frame Disabled {
                n2464 = property on="Material Save" class="Bool"("DisabledEnum"=T30."Enabled" ("Disabled")) -> ()  [unwired: 2 in, 2 out]
              }
              frame Enabled {
              }
            }
            n2465 = property on="Material Copy" class="Bool"("DisabledEnum"=T30."Enabled" ("Disabled")) -> ()  [unwired: 2 in, 2 out]
            "MasterData Image File Path" <- w4113
          }
        }
      }
      event "Material Copy": Value Change {
        n2466 = event-data() -> ()  [unwired: 1 in, 6 out]
        n2467 = local read "Master Data Thermocouple Location"() -> (w4118:picture)
        n2468 = local read "Temp_Host"() -> (w4121:path)
        n2469 = Build Path(base path=w4121, name or relative path="MaterialCopy.jpg") -> (appended path=w4119:path)
        n2470 = call <vilib>:"Picture to Pixmap.vi"("picture"=w4118) -> ("image data"=w4122:T40)  [unwired: 9 in, 1 out]
        n2471 = call <vilib>:"Write JPEG File.vi"("image data"=w4122, "path to JPEG file"=w4119) -> ("error out"=w4117:errorcluster)  [unwired: 8 in, 1 out]
        n2472 = case shown="No Error" w4117 {
          frame No Error {
            n2473 = property on="Material Paste" class="Bool"("DisabledEnum"=T30."Enabled" ("Disabled")) -> ()  [unwired: 2 in, 2 out]
            n2474 = call "Msgbox - Message Handler.vi"("Short Description (When DB Not Available)"="Image Copied", "Description (When DB Not Available)"="Current material image copied.t ", "<.?....> Message Code"="<I 503>") -> ("MHandler Error"=w4123:errorcluster)  [unwired: 6 in, 2 out]
            n2475 = local write "MHandler"(w4123) -> ()
          }
          frame Error {
          }
        }
      }
      event "Material Paste": Value Change {
        n2476 = event-data() -> ()  [unwired: 1 in, 6 out]
        n2477 = local read "Temp_Host"() -> (w4136:path)
        n2478 = Build Path(base path=w4136, name or relative path="MaterialCopy.jpg") -> (appended path=w4132:path)
        n2479 = local write "MasterData Image File Path"(w4132) -> ()
        n2480 = call <vilib>:"Read JPEG File.vi"("path to JPEG file"=w4132) -> ("error out"=w4131:errorcluster, "image data"=w4134:T40)  [unwired: 8 in, 1 out]
        n2481 = call <vilib>:"Draw Flattened Pixmap.vi"("image data"=w4134) -> ("new picture"=w4133:picture)  [unwired: 8 in]
        n2482 = local write "Master Data Thermocouple Location"(w4133) -> ()
        n2483 = Select(t=T30."Disabled and Grayed Out" ("Disabled"), s=w4131, f=T30."Enabled" ("Disabled")) -> (s? t:f=w4130:T30)
        n2484 = disable-structure shown="Disabled" {
          disable-tunnel: w4130 -> [w4137 _]
          frame Disabled {
            n2485 = property on="Material Save" class="Bool"("DisabledEnum"=w4137) -> ()  [unwired: 2 in, 2 out]
          }
          frame Enabled {
          }
        }
      }
      event "Material.Master Data Material", "Master Data Ref Material": Mouse Down? {
        # "<material>_<rev>_<description>.jpg"
        # "<wps/ref>_<rev>.wps"
        # "User Clicks on Material in Parts Details OR Master Data Material OR Master Data Ref Material"
        n2486 = event-data() -> ("CtlRef"=w4139:refnum<vi>)  [unwired: 1 in, 7 out]
        n2487 = local read "DB - Master Data Load"() -> (w4138:bool)
        n2488 = case shown="True" w4138 {
          tunnel: w4139 -> [w4142 w4151]
          frame False {
            n2489 = local read "MasterData\\JPG"() -> (w4140:path)
            n2490 = List Folder(path=w4140, pattern="*.jpg") -> (filenames=w4141:string[])  [unwired: 2 in, 3 out]
            n2491 = local write "Temp Array"(w4141) -> ()
            n2492 = call "String - Extract Unique Headers_.vi"("Array In"=w4141) -> ("Array Out"=w4143:string[])  [unwired: 10 in]
            n2493 = property class="CmbBox"(reference=w4142, "Strings[]"=w4143) -> ()  [unwired: 1 in, 2 out]
          }
          frame True {
            # "Use DB"
            n2494 = property class="CmbBox"(reference=w4151) -> ("Label.Text"=w4150:string)  [unwired: 1 in, 2 out]
            n2495 = case shown="\"Master Data Material\"" w4150 {
              tunnel: [w4154 w4156 w4158] -> w4149
              tunnel: ["SRTRS.MasterData.Material" ("SRTRS.MasterData.SAPMaterial/Material") "SRTRS.MasterData.Material" ("SRTRS.MasterData.SAPMaterial/Material") "SRTRS.MasterData.SAPMaterial" ("SRTRS.MasterData.SAPMaterial/Material")] -> w4145
              frame "Material", Default {
                w4154 = FALSE  # Include Inactive
                # "From Setup Tab"
              }
              frame "Master Data Material" {
                w4156 = TRUE  # Include Inactive
                # "From Master Data Tab"
              }
              frame "Master Data Ref Material" {
                w4158 = FALSE  # Include Inactive
                # "From Master Data Tab"
              }
            }
            n2496 = local read "Logon"() -> (w4148:T21)
            n2497 = Unbundle By Name(w4148) -> ("LanguageID"=w4147:string)
            n2498 = call "DB - [MasterData].[Material].vi"("DB - Master Data Material Enum"=DB_-_Master_Data_Material_Enum."SELECT [MaterialNo]", "Include Inactive"=w4149, "SRTRS.MasterData.SAPMaterial/Material"=w4145, "[LanguageId]"=w4147, "Update [ShortDescription] to Cluster"=TRUE, "CmbBox Refnum"=w4151) -> ()  [unwired: 5 in, 5 out]
          }
        }
        n2499 = event-data() -> ()  [unwired: 2 in, 1 out]
      }
      event "Material.Master Data Material": Value Change {
        n2500 = event-data() -> ("CtlRef"=w4168:refnum<vi>)  [unwired: 1 in, 5 out]
        n2501 = property class="CmbBox"(reference=w4168) -> ("Label.Text"=w4161:string, "Value"=w4160:string)  [unwired: 1 in, 2 out]
        n2502 = case shown="\"Master Data Material\"" w4161 {
          tunnel: [w4206 w4219] -> w4165
          tunnel: [w4205 w4218] -> w4164
          tunnel: [w4204 w4217] -> w4163
          tunnel: [w4203 w4216] -> w4166
          tunnel: w4160 -> [w4197 w4211]
          tunnel: [w4198 w4215] -> w4162
          tunnel: [w4192 w4207] -> w4159
          frame "Material", Default {
            w4192 = TRUE  # Always Update Rev Combo Box
            w4198 = FALSE  # Include Inactive
            # "Item Details.Material"
            n2503 = control-ref of="Material Buffer"() -> (w4202:refnum<vi>)
            n2504 = property class="Clust (strict)"(reference=w4202) -> (reference out=w4199:refnum<vi>, "Value"=w4201:T12)  [unwired: 1 in, 1 out]
            n2505 = Empty String/Path?(string/path=w4197) -> (empty?=w4196:bool)
            n2506 = Bundle By Name(cluster=w4201, "Master Data Material"=w4197) -> (w4200:T12)
            n2507 = control-ref of="Revision"() -> (w4206:refnum<vi>)
            n2508 = control-ref of="Setup Thermocouple Location"() -> (w4204:refnum<vi>)
            n2509 = control-ref of="Material Description"() -> (w4205:refnum<vi>)
            n2510 = Select(t=T30."Disabled and Grayed Out" ("Disabled"), s=w4196, f=T30."Enabled" ("Disabled")) -> (s? t:f=w4195:T30)
            n2511 = property on="SAPMaterial Description (Long) Setup Tab" class="Bool"("DisabledEnum"=w4195) -> ()  [unwired: 2 in, 2 out]
            n2512 = property class="Clust (strict)"(reference=w4199, "Value"=w4200) -> (reference out=w4203:refnum<vi>)  [unwired: 1 in, 1 out]
          }
          frame "Master Data Material" {
            w4215 = TRUE  # Include Inactive
            # "Only allow update of rev ComboBox if nothing in Rev"
            # "Master.Master Data Material"
            n2513 = Empty String/Path?(string/path=w4211) -> (empty?=w4214:bool)
            n2514 = control-ref of="Master Data Thermocouple Location"() -> (w4217:refnum<vi>)
            n2515 = local read "Master Data Ref Material"() -> (w4208:string)
            n2516 = control-ref of="Material"() -> (w4216:refnum<vi>)
            n2517 = control-ref of="Master Data Material Description"() -> (w4218:refnum<vi>)
            n2518 = control-ref of="Master Data Rev"() -> (w4219:refnum<vi>)
            n2519 = Select(t=T30."Disabled and Grayed Out" ("Disabled"), s=w4214, f=T30."Enabled" ("Disabled")) -> (s? t:f=w4210:T30)
            n2520 = property on="SAPMaterial Description (Long) Master Data Tab" class="Bool"("DisabledEnum"=w4210) -> ()  [unwired: 2 in, 2 out]
            n2521 = property on="Material Save" class="Bool"("DisabledEnum"=w4210) -> ()  [unwired: 2 in, 2 out]
            n2522 = String Length(string=w4208) -> (length=w4209:i32)
            n2523 = Equal To 0?(x=w4209) -> (x = 0?=w4207:bool)
          }
        }
        n2524 = local read "DB - Master Data Load"() -> (w4167:bool)
        n2525 = case shown="True" w4167 {
          tunnel: w4165 -> [w4174 w4179]
          tunnel: w4160 -> [w4171 _]
          tunnel: w4166 -> [_ w4180]
          tunnel: w4164 -> [w4170 _]
          tunnel: w4163 -> [w4169 _]
          tunnel: w4162 -> [_ w4178]
          tunnel: w4161 -> [_ w4177]
          tunnel: w4159 -> [_ w4176]
          frame False {
            n2526 = local read "Temp Array"() -> (w4175:string[])
            n2527 = call "String - Extract _Body_.vi"("Temp Array"=w4175, "<wps>"=w4171) -> ("<rev>"=w4173:string[])  [unwired: 9 in]
            n2528 = property class="CmbBox"(reference=w4174, "Strings[]"=w4173, "Val(Sgnl)"="") -> ()  [unwired: 1 in, 2 out]
            n2529 = invoke class="Str" method="Reinit To Default"(reference=w4170) -> ()  [unwired: 2 in, 3 out]
            n2530 = invoke class="Pict" method="Reinit To Default"(reference=w4169) -> ()  [unwired: 2 in, 3 out]
          }
          frame True {
            # "Use DB"
            n2531 = case shown="True" w4176 {
              tunnel: w4180 -> [_ w4191]
              tunnel: w4179 -> [_ w4189]
              tunnel: w4178 -> [_ w4187]
              tunnel: w4177 -> [_ w4182]
              frame False {
                # "Something in Ref. Don't do anything"
              }
              frame True {
                # "Updates Picture"
                # "We will update the [ShortDescription] later during Revision Toggle.\nActually no problem updating here also, but easier to debug code if we\nupdate only in one location."
                # "Updates Rev ComboBox"
                # "Nothing in Ref"
                n2532 = local read "Logon"() -> (w4186:T21)
                n2533 = Unbundle By Name(w4186) -> ("LanguageID"=w4185:string)
                n2534 = call "DB - [MasterData].[Material].vi"("DB - Master Data Material Enum"=DB_-_Master_Data_Material_Enum."SELECT [MaterialRev]", "Include Inactive"=w4187, "[LanguageId]"=w4185, "Update [ShortDescription] to Cluster"=FALSE, "Clust Refnum"=w4191, "CmbBox Refnum"=w4189) -> ("SUMMARY"=w4181:errorcluster)  [unwired: 5 in, 4 out]
                n2535 = local write "DB"(w4181) -> ()
                n2536 = property class="CmbBox"(reference=w4189, "Value"="") -> (error out=w4183:errorcluster)  [unwired: 1 in, 1 out]
                n2537 = property on="Revision Toggle" class="Str"(error in=w4183, "Val(Sgnl)"=w4182) -> ()  [unwired: 1 in, 2 out]
              }
            }
          }
        }
      }
      event "Master Data Ref Material": Value Change {
        # "NA"
        # "COPY MasterData.SAPMaterial.MaterialNo and ShortDescription TO\nMasterData.Material.MaterialNo and Description Controls"
        n2538 = event-data() -> ("CtlRef"=w4222:refnum<vi>)  [unwired: 1 in, 5 out]
        n2539 = property class="CmbBox" props=["Label", "Text", "Value"](reference=w4222) -> ("Value"=w4221:string)  [unwired: 1 in, 3 out]
        n2540 = Empty String/Path?(string/path=w4221) -> (empty?=w4220:bool)
        n2541 = case shown="False" w4220 {
          tunnel: w4221 -> [w4229 _]
          frame False {
            # "Copies Ref Material to Material"
            # "Get Rev"
            n2542 = control-ref of="Master Data Material"() -> (w4226:refnum<vi>)
            n2543 = control-ref of="Material"() -> (w4232:refnum<vi>)
            n2544 = Empty String/Path?(string/path=w4229) -> (empty?=w4235:bool)
            n2545 = property class="Clust (strict)"(reference=w4232) -> (reference out=w4231:refnum<vi>, "Value"=w4230:T12)  [unwired: 1 in, 1 out]
            n2546 = property class="CmbBox"(reference=w4226) -> ("Label.Text"=w4225:string)  [unwired: 1 in, 2 out]
            n2547 = Select(t=T30."Disabled and Grayed Out" ("Disabled"), s=w4235, f=T30."Enabled" ("Disabled")) -> (s? t:f=w4223:T30)
            n2548 = Bundle By Name(cluster=w4230, "Master Data Material"=w4229, "Master Data Rev"="") -> (w4228:T12)
            n2549 = property on="SAPMaterial Description (Long) Master Data Tab" class="Bool"("DisabledEnum"=w4223) -> ()  [unwired: 2 in, 2 out]
